vi "Build Context Menu.vi"(0 "NotifyIcon in":refnum<class "NotifyIcon.lvclass">, 11 "error in (no error)":errorcluster) -> (4 "NotifyIcon out":refnum<class "NotifyIcon.lvclass">, 15 "error out":errorcluster)   [LabVIEW 2016]
doc: "This VI demonstrates how to build the context menu using the NotifyIcon Class member VIs.\n\n\nStinus Olsen\nCIM Industrial Systems A/S\n22. Feb. 2011 15:03\nmailto: seo@cim.as"
uses:
  NotifyIcon.lvclass
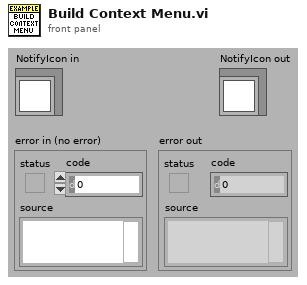
[diagram p1: front panel]
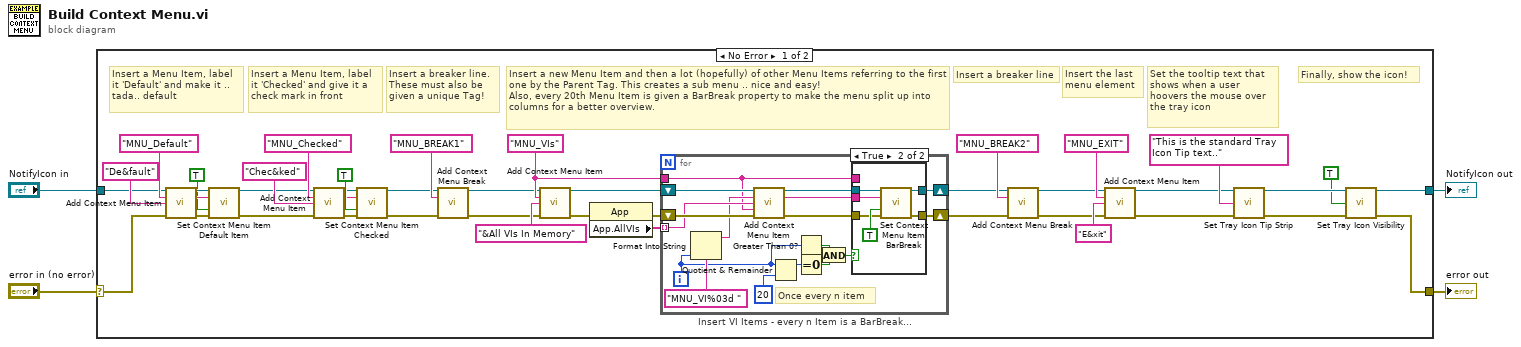
[diagram p0: block diagram]
diagram:
  n1 = case shown="No Error" "error in (no error)" {
    selector: "error in (no error)" -> [w26 w73]
    tunnel: [w41 w73] -> w3
    tunnel: [w42 w72] -> w1
    tunnel: "NotifyIcon in" -> [w27 w72]
    frame No Error {
      w40 = "MNU_VIs" ("Node Tag")
      # "Finally, show the icon!"
      # "Set the tooltip text that\nshows when a user \nhoovers the mouse over\nthe tray icon"
      # "Insert the last\nmenu element"
      # "Insert a breaker line"
      # "Insert a new Menu Item and then a lot (hopefully) of other Menu Items referring to the first one by the Parent Tag. This creates a sub menu .. nice and easy!\nAlso, every 20th Menu Item is given a BarBreak property to make the menu split up into columns for a better overview."
      # "Insert a breaker line.\nThese must also be given a unique Tag!"
      # "Insert a Menu Item, label it 'Checked' and give it a check mark in front"
      # "Insert a Menu Item, label it 'Default' and make it ..tada.. default"
      n2 = call "Add Context Menu Item.vi"("NotifyIcon in"=w27, "Item Tag"="MNU_Default" ("Node Tag"), "Item Text"="De&fault" ("Node Text"), "error in (no error)"=w26) -> ("NotifyIcon out"=w24:refnum<class "NotifyIcon.lvclass">, "dub Item Tag"=w23:string, "error out"=w25:errorcluster)  [unwired: 2 in, 7 out]
      n3 = call "Set Context Menu Item Default Item.vi"("NotifyIcon in"=w24, "Item Tag"=w23, "Default Item (False)"=TRUE, "error in (no error)"=w25) -> ("NotifyIcon out"=w15:refnum<class "NotifyIcon.lvclass">, "error out"=w14:errorcluster)  [unwired: 10 out]
      n4 = call "Add Context Menu Item.vi"("NotifyIcon in"=w15, "Item Tag"="MNU_Checked" ("Node Tag"), "Item Text"="Chec&ked" ("Node Text"), "error in (no error)"=w14) -> ("NotifyIcon out"=w19:refnum<class "NotifyIcon.lvclass">, "dub Item Tag"=w20:string, "error out"=w18:errorcluster)  [unwired: 2 in, 7 out]
      n5 = call "Set Context Menu Item Checked.vi"("NotifyIcon in"=w19, "Item Tag"=w20, "Checked (False)"=TRUE, "error in (no error)"=w18) -> ("NotifyIcon out"=w12:refnum<class "NotifyIcon.lvclass">, "error out"=w11:errorcluster)  [unwired: 10 out]
      n6 = call "Add Context Menu Break.vi"("NotifyIcon in"=w12, "Item Tag"="MNU_BREAK1" ("Node Tag"), "error in (no error)"=w11) -> ("NotifyIcon out"=w9:refnum<class "NotifyIcon.lvclass">, "error out"=w10:errorcluster)  [unwired: 2 in, 9 out]
      n7 = call "Add Context Menu Item.vi"("NotifyIcon in"=w9, "Item Tag"=w40, "Item Text"="&All VIs In Memory" ("String text"), "error in (no error)"=w10) -> ("NotifyIcon out"=w33:refnum<class "NotifyIcon.lvclass">, "error out"=w31:errorcluster)  [unwired: 2 in, 8 out]
      n8 = property class="App"(error in=w31) -> (error out=w32:errorcluster, "App.AllVIs"=w30:string[])  [unwired: 1 in, 1 out]
      n9 = for "Insert VI Items - every n Item is a BarBreak..." {
        shift-right: [w56] -> w8
        shift-left: w33 -> [w63]
        shift-right: [w55] -> w7
        shift-left: w32 -> [w62]
        tunnel: w40 -> [w53]
        tunnel: w30 -> [w60] mode=indexing
        i -> [w50]
        # "Once every n item"
        n10 = Format Into String(format string="MNU_VI%03d " ("string"), w50) -> (resulting string=w54:string)  [unwired: 2 in, 1 out]
        n11 = call "Add Context Menu Item.vi"("NotifyIcon in"=w63, "Item Tag"=w54, "Item Text"=w60, "Parent Item Tag (\"\")"=w53, "error in (no error)"=w62) -> ("NotifyIcon out"=w58:refnum<class "NotifyIcon.lvclass">, "dub Item Tag"=w52:string, "error out"=w59:errorcluster)  [unwired: 1 in, 7 out]
        n12 = Quotient & Remainder(x=w50, y=20 ("n")) -> (x-y*floor(x/y)=w51:i32)  [unwired: 1 out]
        n13 = Greater Than 0?(x=w50) -> (x > 0?=w49:bool)
        n14 = Equal To 0?(x=w51) -> (x = 0?=w48:bool)
        n15 = And(x=w49, y=w48) -> (x .and. y?=w47:bool)
        n16 = case shown="True" w47 {
          tunnel: w59 -> [w64 w67]
          tunnel: w58 -> [w65 w68]
          tunnel: [w65 w69] -> w56
          tunnel: [w64 w70] -> w55
          tunnel: w53 -> [_ _]
          tunnel: w52 -> [_ w66]
          frame False {
          }
          frame True {
            n17 = call "Set Context Menu Item BarBreak.vi"("NotifyIcon in"=w68, "Item Tag"=w66, "BarBreak (False)"=TRUE, "error in (no error)"=w67) -> ("NotifyIcon out"=w69:refnum<class "NotifyIcon.lvclass">, "error out"=w70:errorcluster)  [unwired: 10 out]
          }
        }
      }
      n18 = call "Add Context Menu Break.vi"("NotifyIcon in"=w8, "Item Tag"="MNU_BREAK2" ("Node Tag"), "error in (no error)"=w7) -> ("NotifyIcon out"=w6:refnum<class "NotifyIcon.lvclass">, "error out"=w5:errorcluster)  [unwired: 2 in, 9 out]
      n19 = call "Add Context Menu Item.vi"("NotifyIcon in"=w6, "Item Tag"="MNU_EXIT" ("Node Tag"), "Item Text"="E&xit" ("String text"), "error in (no error)"=w5) -> ("NotifyIcon out"=w35:refnum<class "NotifyIcon.lvclass">, "error out"=w34:errorcluster)  [unwired: 2 in, 8 out]
      n20 = call "Set Tray Icon Tip Strip.vi"("NotifyIcon in"=w35, "Icon Tip Strip Text"="This is the standard Tray Icon Tip text.." ("Node Tag"), "error in (no error)"=w34) -> ("NotifyIcon out"=w45:refnum<class "NotifyIcon.lvclass">, "error out"=w44:errorcluster)  [unwired: 11 out]
      n21 = call "Set Tray Icon Visibility.vi"("NotifyIcon in"=w45, "Show Tray Icon"=TRUE, "error in (no error)"=w44) -> ("NotifyIcon out"=w42:refnum<class "NotifyIcon.lvclass">, "error out"=w41:errorcluster)  [unwired: 11 out]
    }
    frame Error {
    }
  }
  "error out" <- w3
  "NotifyIcon out" <- w1
